vi "ListDevices.vi"() -> ()   [LabVIEW 2014, in "LVTiePie.lvlib"]
uses:
  LVTiePie.lvlib
panel:
  in  "error in (no error)":errorcluster
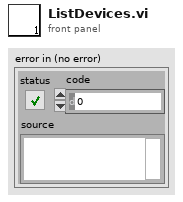
[diagram p1: front panel]
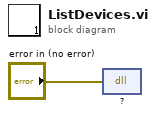
[diagram p0: block diagram]
diagram:
  n1 = dll-call lib="?" fn="?"(error in="error in (no error)") -> ()  [unwired: 3 in, 2 out]
